vi "BRig_RT__Case_Exp__State_Cue__v3.vi"(0 "input_dataCurrent":u16[](array[numeric]), 1 "input_dataTrial":u16[][](array[numeric]), 3 "input_dataExp":u16[](array[numeric]), 4 "input_Cue2":bool, 5 "input_arrTrig":bool[](array[boolean]), 6 "input_state":T1, 8 "I_lick":bool) -> (7 "output_l2_laserOn":bool, 9 "output_l2_laserEvent":bool, 10 "output_SelectionState":bool, 11 "output_l1_laserOn":bool, 12 "output_state":T1, 13 "output_l1_laserEvent":bool, 14 "output_dataCurrent":u16[](array[numeric]), 15 "output_dataTrial":u16[][](array[numeric]), 17 "output_CueLed":bool, 18 "output_Audio_L":bool, 19 "output_Audio_R":bool)   [LabVIEW 2014]
uses:
  myRIO_BRig_RT__Case_Exp_stateList.ctl
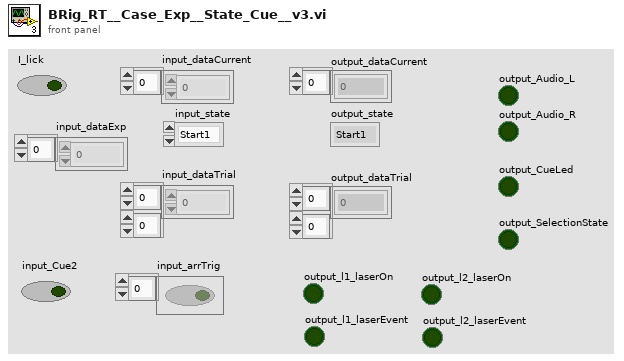
[diagram p1: front panel]
types:
  T1 = typedef "myRIO_BRig_RT__Case_Exp_stateList.ctl" = enum16{"Start1", "Start2", "Start3", "saveSettings1", "saveSettings2", "saveSettings3", "saveSettings4", "saveSettings_LC_ENL_l1", "saveSettings_LC_ENL_l2", "saveSettings_LC_Cue_l1", "saveSettings_LC_Cue_l2", "saveSettings6_LC_l1_Other", "SaveSettings6_LC_l2_Other", "setSettings_Audio", "setSettings_Laser", "initBlock_pre", "initBlock", "initBlock2", "initBlock_post", "initTrial_pre", "initTrial", "initTrial2", "initTrial3", "initTrial4", "initTrial_LC_ENL1", "initTrial_LC_Cue1", "initTrial_LC_Cue1_2", "initTrial_LC_Sel", "initTrial_post", "ENL1_pre", "ENL1", "ENL1_post", "ENL1Penalty_pre", "ENL1Penalty", "ENL2_pre", "ENL2", "ENL2Penalty_pre", "ENL2Penalty", "Cue1_pre", "Cue1", "Cue1_post", "Cue1Penalty_pre", "Cue1Penalty", "Cue2_pre", "Cue2", "Cue2Penalty_pre", "Cue2Penalty", "Selection_pre", "Selection", "Select_post", "SelectReward_pre", "SelectReward", "SelectRewardPost_pre", "SelectRewardPost", "SelectWrong_pre", "SelectWrong", "SelectWrong_post", "SelectTimeout_pre", "SelectTimeout", "SelectTimeout_post", "endTrial_pre", "endTrial1", "endTrial2", "endTrial3", "endTrial_post", "endBlock_pre", "endBlock", "endBlock_post", "endExp", "commConnect", "commUpload_pre", "commUpload_dataBlock", "commUpload_dataCurrent", "commUpload_dataExp", "commUpload_dataLC", "commUpload_dataTrial", "commUpload_post", "saveData_pre", "saveData_dataBlock", "saveData_dataCurrent", "saveData_dataExp", "saveData_dataLC", "saveData_dataTrial", "saveData_post", "empty_endBlock1", "empty_endBlock2", "empty_endTrial1", "empty_endTrial2", "empty_endTrial3", "empty_endTrial4", "empty_endTrial5", "dummyState", "dummyState_endBlock", "FreeReward_pre", "FreeReward", "FreeRewardPost_pre", "FreeRewardPost"}
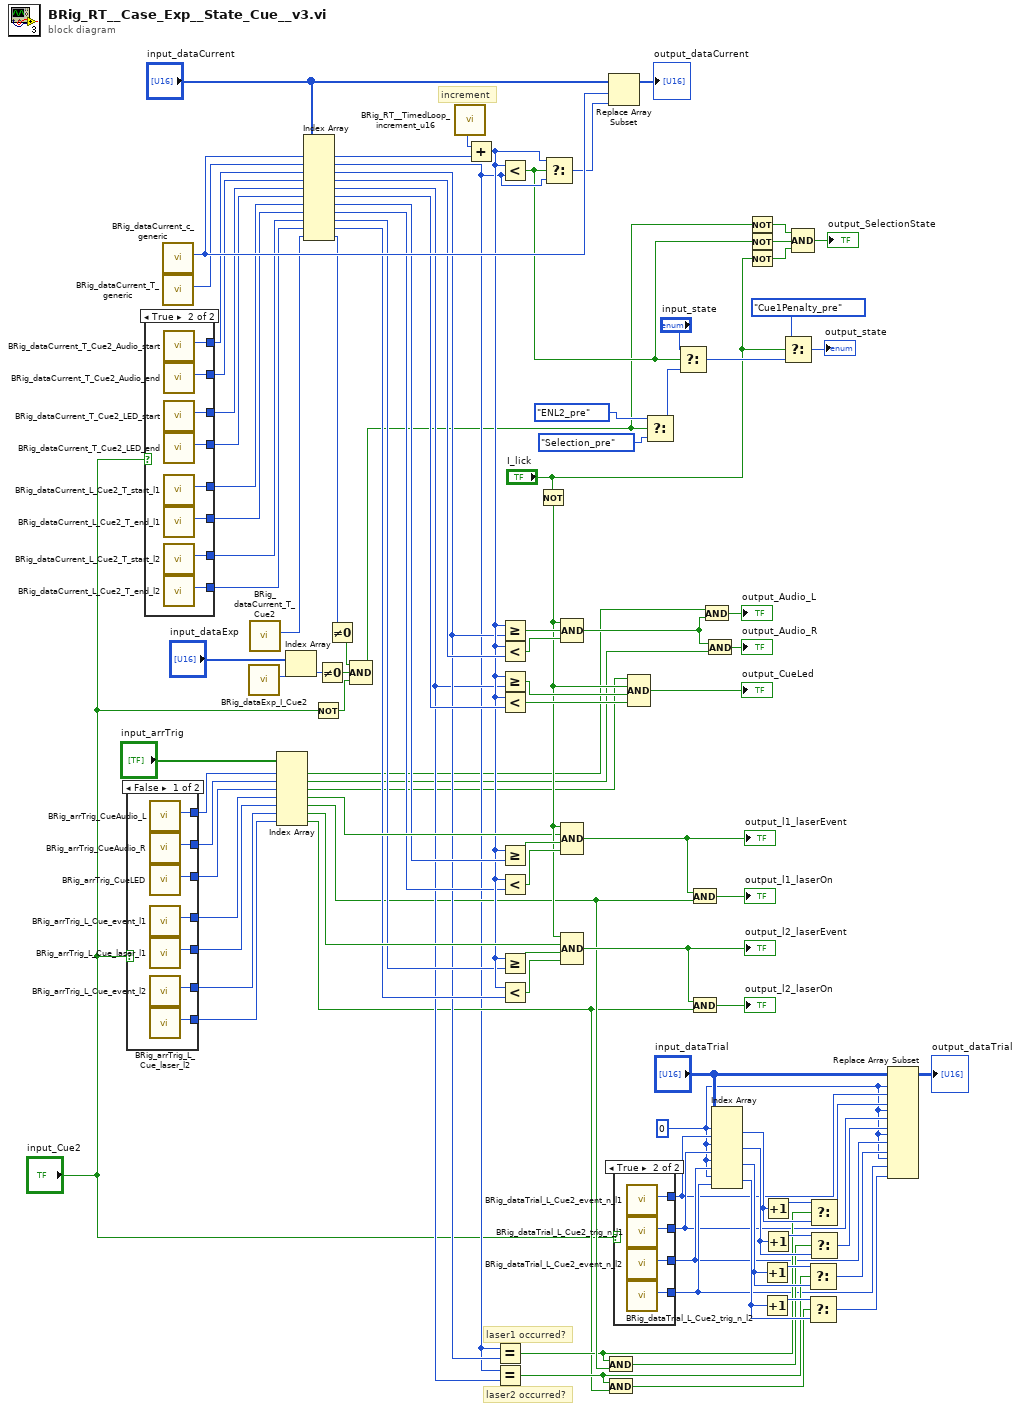
[diagram p0: block diagram]
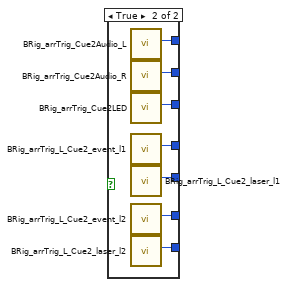
[diagram p2: hidden frame]
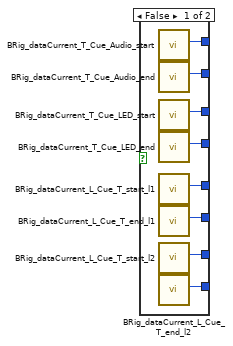
[diagram p3: hidden frame]
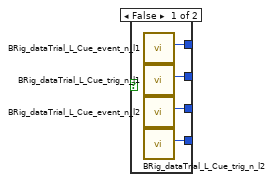
[diagram p4: hidden frame]
diagram:
  w23 = 0
  # "laser2 occurred?"
  # "laser1 occurred?"
  # "increment"
  n1 = case shown="False" "input_Cue2" {
    tunnel: [w110 w117] -> w87
    tunnel: [w109 w115] -> w86
    tunnel: [w108 w116] -> w85
    tunnel: [w107 w114] -> w84
    tunnel: [w106 w113] -> w3
    tunnel: [w105 w112] -> w2
    tunnel: [w104 w111] -> w1
    frame False {
      n2 = call "BRig_arrTrig_CueAudio_L.vi"() -> ("output_CueAudio_L"=w106:i32)  [unwired: 11 in]
      n3 = call "BRig_arrTrig_CueAudio_R.vi"() -> ("output_CueAudio_R"=w105:i32)  [unwired: 11 in]
      n4 = call "BRig_arrTrig_CueLED.vi"() -> ("output_CueLED"=w104:i32)  [unwired: 11 in]
      n5 = call "BRig_arrTrig_L_Cue_event_l1.vi"() -> ("output_L_Cue_event_l1"=w110:i32)  [unwired: 11 in]
      n6 = call "BRig_arrTrig_L_Cue_laser_l1.vi"() -> ("output_L_Cue_laser_l1"=w108:i32)  [unwired: 11 in]
      n7 = call "BRig_arrTrig_L_Cue_event_l2.vi"() -> ("output_L_Cue_event_l2"=w109:i32)  [unwired: 11 in]
      n8 = call "BRig_arrTrig_L_Cue_laser_l2.vi"() -> ("output_L_Cue_laser_l2"=w107:i32)  [unwired: 11 in]
    }
    frame True {
      n9 = call "BRig_arrTrig_Cue2Audio_L.vi"() -> ("output_Cue2Audio_L"=w113:i32)  [unwired: 11 in]
      n10 = call "BRig_arrTrig_Cue2Audio_R.vi"() -> ("output_Cue2Audio_R"=w112:i32)  [unwired: 11 in]
      n11 = call "BRig_arrTrig_Cue2LED.vi"() -> ("output_Cue2LED"=w111:i32)  [unwired: 11 in]
      n12 = call "BRig_arrTrig_L_Cue2_event_l1.vi"() -> ("output_L_Cue2_event_l1"=w117:i32)  [unwired: 11 in]
      n13 = call "BRig_arrTrig_L_Cue2_laser_l1.vi"() -> ("output_L_Cue2_laser_l1"=w116:i32)  [unwired: 11 in]
      n14 = call "BRig_arrTrig_L_Cue2_event_l2.vi"() -> ("output_L_Cue2_event_l2"=w115:i32)  [unwired: 11 in]
      n15 = call "BRig_arrTrig_L_Cue2_laser_l2.vi"() -> ("output_L_Cue2_laser_l2"=w114:i32)  [unwired: 11 in]
    }
  }
  n16 = case shown="True" "input_Cue2" {
    tunnel: [w125 w133] -> w81
    tunnel: [w124 w132] -> w80
    tunnel: [w123 w131] -> w78
    tunnel: [w122 w130] -> w77
    tunnel: [w121 w129] -> w63
    tunnel: [w120 w128] -> w62
    tunnel: [w119 w127] -> w61
    tunnel: [w118 w126] -> w60
    frame False {
      n17 = call "BRig_dataCurrent_T_Cue_Audio_start.vi"() -> ("output_T_Cue_Audio_start"=w125:i32)  [unwired: 11 in]
      n18 = call "BRig_dataCurrent_T_Cue_Audio_end.vi"() -> ("output_T_Cue_Audio_end"=w124:i32)  [unwired: 11 in]
      n19 = call "BRig_dataCurrent_T_Cue_LED_start.vi"() -> ("output_T_Cue_LED_start"=w123:i32)  [unwired: 11 in]
      n20 = call "BRig_dataCurrent_T_Cue_LED_end.vi"() -> ("output_T_Cue_LED_end"=w122:i32)  [unwired: 11 in]
      n21 = call "BRig_dataCurrent_L_Cue_T_start_l1.vi"() -> ("outputL_Cue_T_start_l1"=w121:i32)  [unwired: 11 in]
      n22 = call "BRig_dataCurrent_L_Cue_T_end_l1.vi"() -> ("output_L_Cue_T_end_l1"=w120:i32)  [unwired: 11 in]
      n23 = call "BRig_dataCurrent_L_Cue_T_start_l2.vi"() -> ("output_L_Cue_T_start_l2"=w119:i32)  [unwired: 11 in]
      n24 = call "BRig_dataCurrent_L_Cue_T_end_l2.vi"() -> ("output_L_Cue_T_end_l2"=w118:i32)  [unwired: 11 in]
    }
    frame True {
      n25 = call "BRig_dataCurrent_T_Cue2_Audio_start.vi"() -> ("output_T_Cue2_Audio_start"=w133:i32)  [unwired: 11 in]
      n26 = call "BRig_dataCurrent_T_Cue2_Audio_end.vi"() -> ("output_T_Cue2_Audio_end"=w132:i32)  [unwired: 11 in]
      n27 = call "BRig_dataCurrent_T_Cue2_LED_start.vi"() -> ("output_T_Cue2_LED_start"=w131:i32)  [unwired: 11 in]
      n28 = call "BRig_dataCurrent_T_Cue2_LED_end.vi"() -> ("output_T_Cue2_LED_end"=w130:i32)  [unwired: 11 in]
      n29 = call "BRig_dataCurrent_L_Cue2_T_start_l1.vi"() -> ("outputL_Cue2_T_start_l1"=w129:i32)  [unwired: 11 in]
      n30 = call "BRig_dataCurrent_L_Cue2_T_end_l1.vi"() -> ("output_L_Cue2_T_end_l1"=w128:i32)  [unwired: 11 in]
      n31 = call "BRig_dataCurrent_L_Cue2_T_start_l2.vi"() -> ("output_L_Cue2_T_start_l2"=w127:i32)  [unwired: 11 in]
      n32 = call "BRig_dataCurrent_L_Cue2_T_end_l2.vi"() -> ("output_L_Cue2_T_end_l2"=w126:i32)  [unwired: 11 in]
    }
  }
  n33 = call "BRig_dataCurrent_c_generic.vi"() -> ("output_count_generic"=w83:i32)  [unwired: 11 in]
  n34 = call "BRig_dataCurrent_T_generic.vi"() -> ("output_T_generic"=w82:i32)  [unwired: 11 in]
  n35 = call "BRig_dataExp_I_Cue2.vi"() -> ("output_I_Cue2"=w20:i32)  [unwired: 11 in]
  n36 = call "BRig_dataCurrent_T_Cue2.vi"() -> ("output_T_Cue2"=w22:i32)  [unwired: 11 in]
  n37 = Index Array(array="input_arrTrig", index #1=w3, index #2=w2, index #3=w1, index #4=w87, index #5=w85, index #6=w86, index #7=w84) -> (element #1=w24:bool, element #2=w26:bool, element #3=w27:bool, element #4=w65:bool, element #5=w38:bool, element #6=w64:bool, element #7=w35:bool)
  n38 = Index Array(array="input_dataExp", index=w20) -> (element=w19:u16)
  n39 = Index Array(array="input_dataCurrent", index #1=w83, index #2=w82, index #3=w81, index #4=w80, index #5=w78, index #6=w77, index #7=w63, index #8=w62, index #9=w61, index #10=w60, index #11=w22) -> (element #1=w79:u16, element #2=w28:u16, element #3=w40:u16, element #4=w71:u16, element #5=w39:u16, element #6=w70:u16, element #7=w59:u16, element #8=w57:u16, element #9=w56:u16, element #10=w55:u16, element #11=w18:u16)
  n40 = Not(x="input_Cue2") -> (.not. x?=w12:bool)
  n41 = Not Equal To 0?(x=w19) -> (x != 0?=w14:bool)
  n42 = Not Equal To 0?(x=w18) -> (x != 0?=w13:bool)
  n43 = Compound Arithmetic op=AND(w13, w14, w12) -> (w9:bool)
  n44 = call "BRig_RT__TimedLoop_increment_u16.vi"() -> ("output_increment__u16"=w100:u16)  [unwired: 11 in]
  n45 = Add(x=w100, y=w79) -> (x+y=w58:u16)
  n46 = Equal?(x=w28, y=w40) -> (x = y?=w37:bool)
  n47 = Equal?(x=w28, y=w39) -> (x = y?=w36:bool)
  n48 = Less?(x=w58, y=w28) -> (x < y?=w10:bool)
  n49 = Greater Or Equal?(x=w58, y=w40) -> (x >= y?=w75:bool)
  n50 = Less?(x=w58, y=w71) -> (x < y?=w76:bool)
  n51 = Greater Or Equal?(x=w58, y=w39) -> (x >= y?=w73:bool)
  n52 = Less?(x=w58, y=w70) -> (x < y?=w72:bool)
  n53 = Greater Or Equal?(x=w58, y=w59) -> (x >= y?=w98:bool)
  n54 = Less?(x=w58, y=w57) -> (x < y?=w99:bool)
  n55 = Greater Or Equal?(x=w58, y=w56) -> (x >= y?=w91:bool)
  n56 = Less?(x=w58, y=w55) -> (x < y?=w90:bool)
  n57 = Not(x="I_lick") -> (.not. x?=w66:bool)
  n58 = Select(t=w58, s=w10, f=w28) -> (s? t:f=w74:u16)
  n59 = Compound Arithmetic op=AND(w66, w75, w76) -> (w25:bool)
  n60 = Compound Arithmetic op=AND(w66, w65, w98, w99) -> (w93:bool)
  "output_l1_laserEvent" <- w93
  n61 = Compound Arithmetic op=AND(w66, w64, w91, w90) -> (w89:bool)
  "output_l2_laserEvent" <- w89
  n62 = And(x=w37, y=w38) -> (x .and. y?=w34:bool)
  n63 = And(x=w36, y=w35) -> (x .and. y?=w33:bool)
  n64 = Replace Array Subset(array="input_dataCurrent", new element=w74, index=w83) -> (→"output_dataCurrent":u16[])
  n65 = case shown="True" "input_Cue2" {
    tunnel: [w137 w138] -> w32
    tunnel: [w136 w139] -> w31
    tunnel: [w135 w140] -> w30
    tunnel: [w134 w141] -> w29
    frame False {
      n66 = call "BRig_dataTrial_L_Cue_event_n_l1.vi"() -> ("output_L_Cue_event_n_l1"=w134:i32)  [unwired: 11 in]
      n67 = call "BRig_dataTrial_L_Cue_trig_n_l1.vi"() -> ("output_L_Cue_trig_n_l1"=w135:i32)  [unwired: 11 in]
      n68 = call "BRig_dataTrial_L_Cue_event_n_l2.vi"() -> ("output_L_Cue_event_n_l2"=w136:i32)  [unwired: 11 in]
      n69 = call "BRig_dataTrial_L_Cue_trig_n_l2.vi"() -> ("output_L_Cue_trig_n_l2"=w137:i32)  [unwired: 11 in]
    }
    frame True {
      n70 = call "BRig_dataTrial_L_Cue2_event_n_l1.vi"() -> ("output_L_Cue2_event_n_l1"=w141:i32)  [unwired: 11 in]
      n71 = call "BRig_dataTrial_L_Cue2_trig_n_l1.vi"() -> ("output_L_Cue2_trig_n_l1"=w140:i32)  [unwired: 11 in]
      n72 = call "BRig_dataTrial_L_Cue2_event_n_l2.vi"() -> ("output_L_Cue2_event_n_l2"=w139:i32)  [unwired: 11 in]
      n73 = call "BRig_dataTrial_L_Cue2_trig_n_l2.vi"() -> ("output_L_Cue2_trig_n_l2"=w138:i32)  [unwired: 11 in]
    }
  }
  n74 = Compound Arithmetic op=AND(w27, w66, w73, w72) -> (→"output_CueLed":bool)
  n75 = Select(t=myRIO_BRig_RT__Case_Exp_stateList."ENL2_pre" ("Enum"), s=w9, f=myRIO_BRig_RT__Case_Exp_stateList."Selection_pre" ("Enum")) -> (s? t:f=w16:T1)
  n76 = Select(t="input_state", s=w10, f=w16) -> (s? t:f=w101:T1)
  n77 = And(x=w93, y=w38) -> (x .and. y?=→"output_l1_laserOn":bool)
  n78 = And(x=w89, y=w35) -> (x .and. y?=→"output_l2_laserOn":bool)
  n79 = And(x=w24, y=w25) -> (x .and. y?=→"output_Audio_L":bool)
  n80 = And(x=w25, y=w26) -> (x .and. y?=→"output_Audio_R":bool)
  n81 = Index Array(array="input_dataTrial", index (row) #1=w23, index (col) #1=w29, index (row) #2=w23, index (col) #2=w30, index (row) #3=w23, index (col) #3=w31, index (row) #4=w23, index (col) #4=w32) -> (element #1=w52:u16, element #2=w48:u16, element #3=w47:u16, element #4=w46:u16)
  n82 = Not(x=w9) -> (.not. x?=w7:bool)
  n83 = Not(x=w10) -> (.not. x?=w8:bool)
  n84 = Not(x="I_lick") -> (.not. x?=w6:bool)
  n85 = Increment(x=w47) -> (x+1=w50:u16)
  n86 = Increment(x=w46) -> (x+1=w49:u16)
  n87 = Increment(x=w52) -> (x+1=w53:u16)
  n88 = Increment(x=w48) -> (x+1=w51:u16)
  n89 = Select(t=myRIO_BRig_RT__Case_Exp_stateList."Cue1Penalty_pre" ("Enum"), s="I_lick", f=w101) -> (s? t:f=→"output_state":T1)
  n90 = Compound Arithmetic op=AND(w7, w8, w6) -> (→"output_SelectionState":bool)
  n91 = Select(t=w50, s=w36, f=w47) -> (s? t:f=w43:u16)
  n92 = Select(t=w49, s=w33, f=w46) -> (s? t:f=w42:u16)
  n93 = Select(t=w53, s=w37, f=w52) -> (s? t:f=w45:u16)
  n94 = Select(t=w51, s=w34, f=w48) -> (s? t:f=w44:u16)
  n95 = Replace Array Subset(array="input_dataTrial", new element #1=w45, index (row) #1=w23, index (col) #1=w29, new element #2=w44, index (row) #2=w23, index (col) #2=w30, new element #3=w43, index (row) #3=w23, index (col) #3=w31, new element #4=w42, index (row) #4=w23, index (col) #4=w32) -> (→"output_dataTrial":u16[][])
